vi "Do Something Else.vi"(8 "error in (no error)":errorcluster, 9 "X":dbl, 10 "Do Something Else Message":string) -> (0 "error out":errorcluster)   [LabVIEW 2019, in "Monedas.lvlib"]
doc: "Send the Do Something Else request to the Module's Main.vi.\n_____\nBased on DQMH Project Template 6.1.0.94."
uses:
  Program Files (x86)/National Instruments/LabVIEW 2019/ProjectTemplates/Source/Delacor/Delacor QMH/Project Template/Libraries/My Singleton Module/Monedas.lvlib
  Do Something Else Argument--cluster.ctl
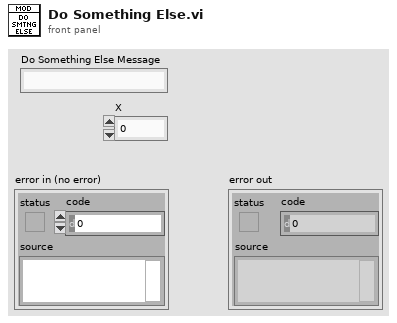
[diagram p1: front panel]
types:
  T1 = typedef "Monedas.lvlib/Do Something Else Argument--cluster.ctl" = cluster{"Do Something Else Msg":string, "X":dbl}
  T2 = typedef "Monedas.lvlib/Request Events--cluster.ctl" = cluster{"Stop Module":refnum<user-event>, "Do Something":refnum<user-event>, "Do Something Else":refnum<user-event>, "Do Something Else and Wait for Reply":refnum<user-event>, "Show Panel":refnum<user-event>, "Hide Panel":refnum<user-event>, "Get Module Execution Status":refnum<user-event>, "Show Diagram":refnum<user-event>}
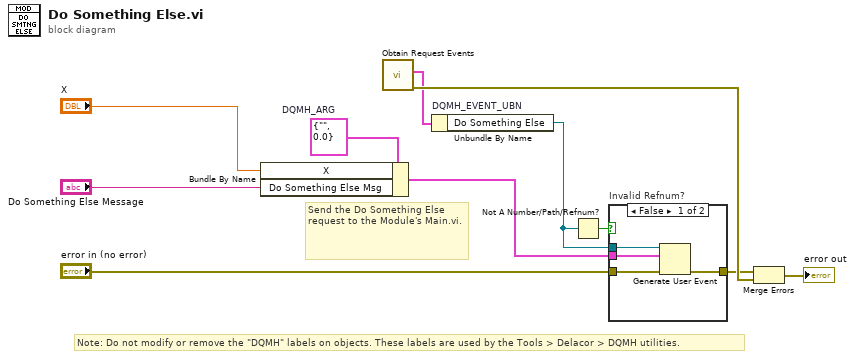
[diagram p0: block diagram]
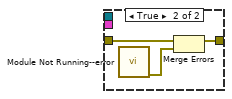
[diagram p2: hidden frame]
diagram:
  w7 = T1 {"Do Something Else Msg"="", "X"=0.0}  # DQMH_ARG
  # "Note: Do not modify or remove the \"DQMH\" labels on objects. These labels are used by the Tools > Delacor > DQMH utilities."
  # "Send the Do Something Else request to the Module's Main.vi."
  n1 = Bundle By Name(cluster=w7, "X"="X", "Do Something Else Msg"="Do Something Else Message") -> (w4:T1)
  n2 = call "Obtain Request Events.vi"() -> ("error out"=w9:errorcluster, "Monedas Request Events"=w8:T2)  [unwired: 10 in]
  n3 = Unbundle By Name "DQMH_EVENT_UBN"(w8) -> ("Do Something Else"=w5:refnum<user-event>)
  n4 = Not A Number/Path/Refnum?(number/path/refnum=w5) -> (NaN/Path/Refnum?=w6:bool)
  n5 = case "Invalid Refnum?" shown="False" w6 {
    tunnel: "error in (no error)" -> [w15 w18]
    tunnel: [w14 w16] -> w1
    tunnel: w4 -> [w13 _]
    tunnel: w5 -> [w12 _]
    frame False {
      n6 = Generate User Event(user event=w12, event data cluster=w13, error in=w15) -> (error out=w14:errorcluster)  [unwired: 1 in, 1 out]
    }
    frame True {
      n7 = call "Module Not Running--error.vi"() -> ("error out"=w17:errorcluster)  [unwired: 11 in]
      n8 = Merge Errors(w18, w17) -> (w16:errorcluster)
    }
  }
  n9 = Merge Errors(w1, w9) -> (→"error out":errorcluster)
